vi "Test Copy Image Greyscale Mask ARGB.vi"(8 "error in (no error)":errorcluster, 11 "Test Case In":refnum<class "01_Image.lvclass">) -> (0 "error out":errorcluster, 3 "Test Case Out":refnum<class "01_Image.lvclass">)   [LabVIEW 2020, in "test.lvlib" / "01_Image.lvclass"]
uses:
  01_Image.lvclass
  C:/Program Files (x86)/National Instruments/LabVIEW 2026/vi.lib/Astemes/LUnit/Test Case.lvclass
  common/Image Size (Integer).ctl
  <vilib>/Astemes/LUnit/Test Case.lvclass/Test Case.ctl
  image/New Image (Greyscale Preallocated).vi
  image/Copy Array to Image (Greyscale).vi
  image/New Image (ARGB Preallocated).vi
  image/Copy Image (ARGB with Greyscale Mask).vi
  4993e8ee-a06a-463a-9684-69129f64d5ce.vi
  image/Copy Array to Image (ARGB).vi
  image/New Image (Greyscale Preallocated).vi/6598b9e0-8a08-46f5-91fd-ca1b87217137.vi
  image/New Image (ARGB Preallocated).vi/3321fa97-f432-4e1e-8db9-a0df79aed21b.vi
  image/ARGB Colour to U32 Pixel Value.vi
  image/Copy Image (ARGB with Greyscale Mask).vi/327a14ae-2acc-4952-87c0-fab6c3cd3da3.vi
  <vilib>/Astemes/LUnit/Core/LUnit Test Case/Private/Append Pass Result.vi
  <vilib>/Astemes/LUnit/Core/LUnit Test Case/Private/Append Fail Result.vi
  4993e8ee-a06a-463a-9684-69129f64d5ce.vi/9c5d11cd-9439-4240-a1ee-d9baace9c924.vi
  <vilib>/Astemes/LUnit/Core/LUnit Test Case/Private/Run In UI.vi
  <vilib>/Utility/error.llb/Clear Errors.vi
  <vilib>/Utility/error.llb/Error Cluster From Error Code.vi
  <vilib>/picture/pixmap.llb/Flatten Pixmap.vi
  image/image.lvlib
  common/common.lvlib
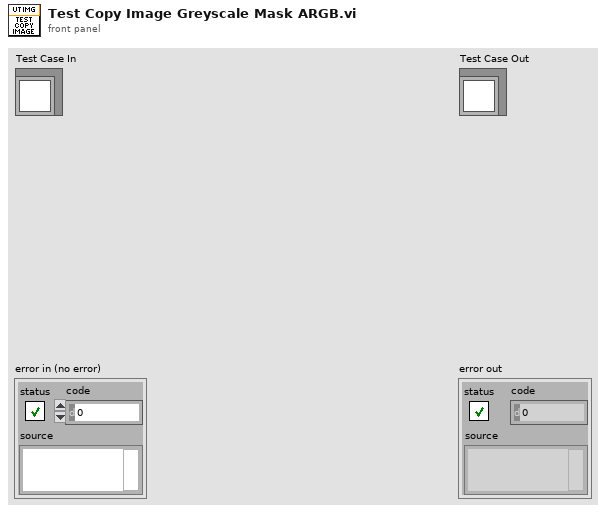
[diagram p1: front panel]
types:
  T1 = typedef "common.lvlib/Image Size (Integer).ctl" = cluster{"Width":u16, "Height":u16}
  T2 = typedef "image.lvlib/ARGB Image.ctl" = refnum<data-value>
  T3 = typedef "image.lvlib/Greyscale Image.ctl" = refnum<data-value>
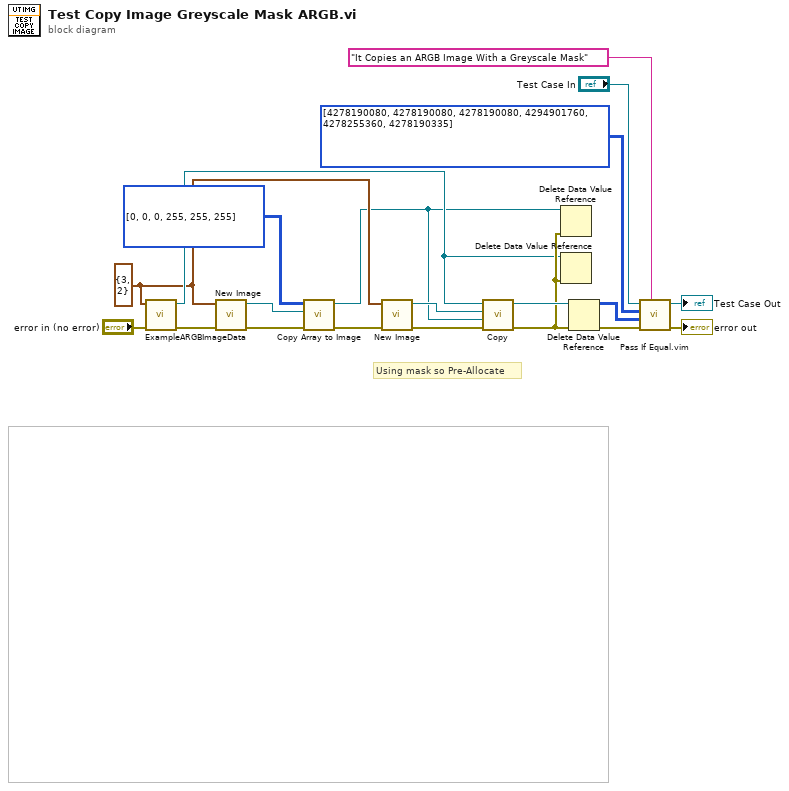
[diagram p0: block diagram]
diagram:
  w7 = T1 {"Width"=3, "Height"=2} ("Preallocated Image Size (Default - 0,0)")
  # "Using mask so Pre-Allocate"
  n1 = call "ExampleARGBImageData.vi"("error in (no error)"="error in (no error)", "Image Size"=w7) -> ("error out"=w11:errorcluster, "Data Value Reference out"=w8:T2)  [unwired: 6 in, 2 out]
  n2 = call-poly "New Image.vi"("error in (no error)"=w11, "Preallocated Image Size (Default 0,0)"=w7) -> ("error out"=w15:errorcluster, "Greyscale Image"=w4:T3)  [unwired: 8 in]
  n3 = call-poly "Copy Array to Image.vi"("error in (no error)"=w15, "Greyscale Destination Image in"=w4, "U8 Greyscale Data"=u8[][] [[0, 0, 0], [255, 255, 255]] ("Source")) -> ("error out"=w6:errorcluster, "Greyscale Destination Image"=w3:T3)  [unwired: 7 in]
  n4 = call-poly "New Image.vi"("error in (no error)"=w6, "Preallocated Image Size (Default: 0,0)"=w7) -> ("error out"=w16:errorcluster, "ARGB Image"=w10:T2)  [unwired: 8 in]
  n5 = call-poly "Copy.vi"("error in (no error)"=w16, "Greyscale Image Mask in"=w3, "ARGB Image Destination in"=w10, "ARGB Image Source in"=w8) -> ("error out"=w9:errorcluster, "ARGB Image Destination"=w13:T2)  [unwired: 6 in]
  n6 = Delete Data Value Reference(data value reference=w3, error in=w9) -> ()  [unwired: 2 out]
  n7 = Delete Data Value Reference(data value reference=w8, error in=w9) -> ()  [unwired: 2 out]
  n8 = Delete Data Value Reference(data value reference=w13, error in=w9) -> (data value=w2:u32[][], error out=w14:errorcluster)
  n9 = call "Pass If Equal.vim"("Description"="It Copies an ARGB Image With a Greyscale Mask", "error in (no error)"=w14, "Actual"=w2, "Expected"=u32[][] [[4278190080, 4278190080, 4278190080], [4294901760, 4278255360, 4278190335]] ("data value"), "LUnit Test Case In"="Test Case In") -> ("error out"=→"error out":errorcluster, "LUnit Test Case Out"=→"Test Case Out":refnum<class "01_Image.lvclass">)  [unwired: 5 in]
